vi "HandleMsg.vi"(0 "reference in":refnum<class "Stand.lvclass">, 5 "message in":T1, 7 "Unhandled in":bool, 11 "error in (no error)":errorcluster) -> (4 "reference out":refnum<class "Stand.lvclass">, 6 "message out":T1, 8 "Unhandled out":bool, 15 "error out":errorcluster)   [LabVIEW 2019, in "Stand.lvclass"]
uses:
  Stand.lvclass
  Device_class/Device.lvclass
  MessageInterface_class/Message.ctl
  MessageInterface_class/MessageInterface.lvclass
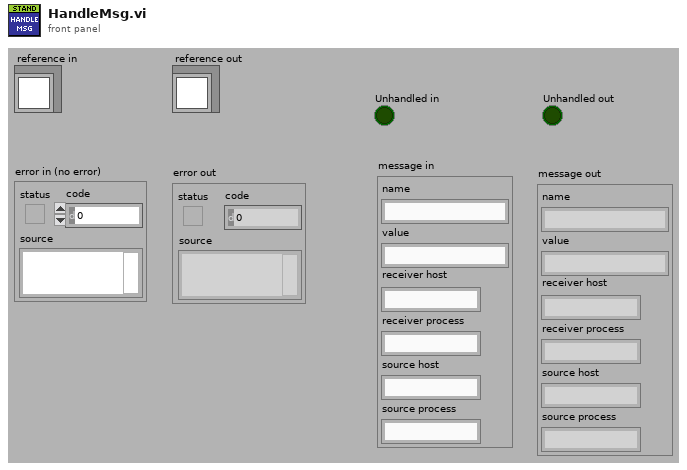
[diagram p1: front panel]
types:
  T1 = typedef "MessageInterface.lvclass/Message.ctl" = cluster{"name":string, "value":string, "receiver host":string, "receiver process":string, "source host":string, "source process":string}
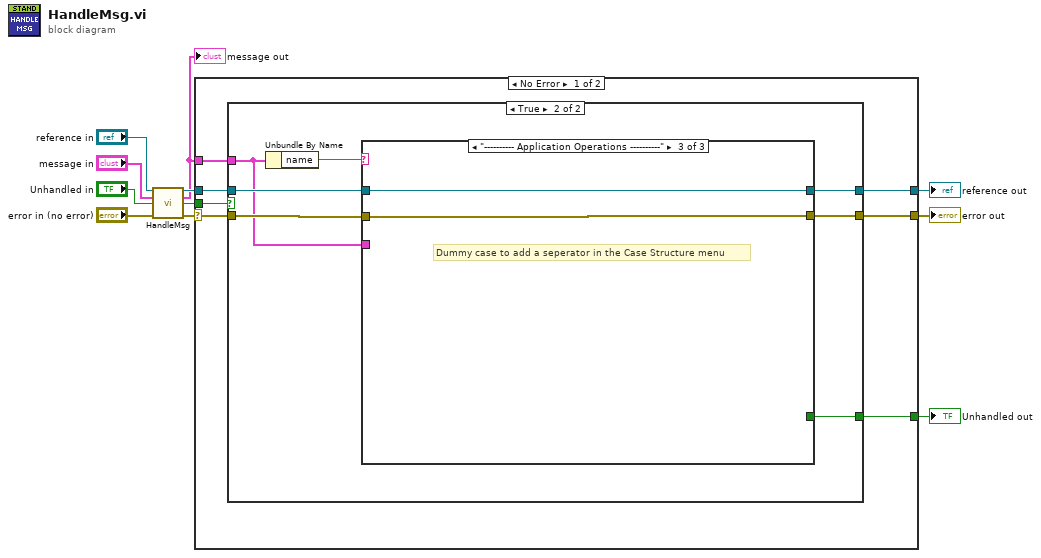
[diagram p0: block diagram]
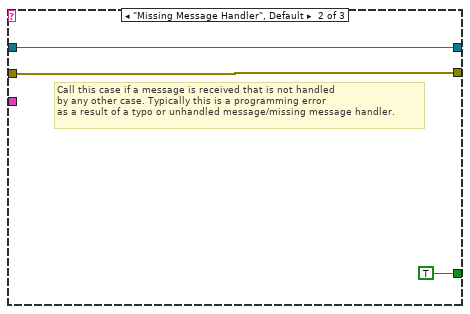
[diagram p4: hidden frame]
diagram:
  n1 = call-parent "HandleMsg.vi"("reference in"="reference in", "message in"="message in", "Unhandled in"="Unhandled in", "error in (no error)"="error in (no error)") -> ("reference out"=w5:refnum<class "Stand.lvclass">, "message out"=w1:T1, "Unhandled out"=w6:bool, "error out"=w7:errorcluster)  [unwired: 8 in]
  "message out" <- w1
  n2 = case shown="No Error" w7 {
    selector: w7 -> [w17 w36]
    tunnel: [w14 w36] -> w4
    tunnel: [w16 w35] -> w3
    tunnel: w5 -> [w18 w35]
    tunnel: w1 -> [w15 _]
    tunnel: [w13 _] -> w2
    tunnel: w6 -> [w12 _]
    frame No Error {
      n3 = case shown="True" w12 {
        tunnel: w18 -> [w20 w27]
        tunnel: w17 -> [w19 w26]
        tunnel: [w20 w25] -> w16
        tunnel: w15 -> [_ w21]
        tunnel: [w19 w23] -> w14
        tunnel: [_ w22] -> w13
        frame False {
        }
        frame True {
          n4 = Unbundle By Name(w21) -> ("name"=w24:string)
          n5 = case shown="\"---------- Application Operations ----------\"" w24 {
            tunnel: [_ TRUE _] -> w22
            tunnel: [w29 w31 w34] -> w25
            tunnel: w27 -> [w29 w31 w34]
            tunnel: [w28 w30 w33] -> w23
            tunnel: w26 -> [w28 w30 w33]
            tunnel: w21 -> [_ _ _]
            frame "", "Idle" {
              # "Idle Case - this case is called after a Timeout on the Get Next Message from Queue VI, if no new messages are present on the queue. This case can be used for housekeeping tasks such as updating the UI."
            }
            frame "Missing Message Handler", Default {
              # "Call this case if a message is received that is not handled \nby any other case. Typically this is a programming error\nas a result of a typo or unhandled message/missing message handler."
            }
            frame "---------- Application Operations ----------" {
              # "Dummy case to add a seperator in the Case Structure menu"
            }
          }
        }
      }
    }
    frame Error {
    }
  }
  "error out" <- w4
  "reference out" <- w3
  "Unhandled out" <- w2
